vi "Auto_Routine_Deposit.vi"(8 "error in (no error)":errorcluster, 10 "Game Piece":T1, 11 "Position":T2=enum."Middle") -> (0 "error out":errorcluster)   [LabVIEW 2020]
uses:
  Arm/ArmPositionPreset.ctl
  Arm/ArmGamePiecePreset.ctl
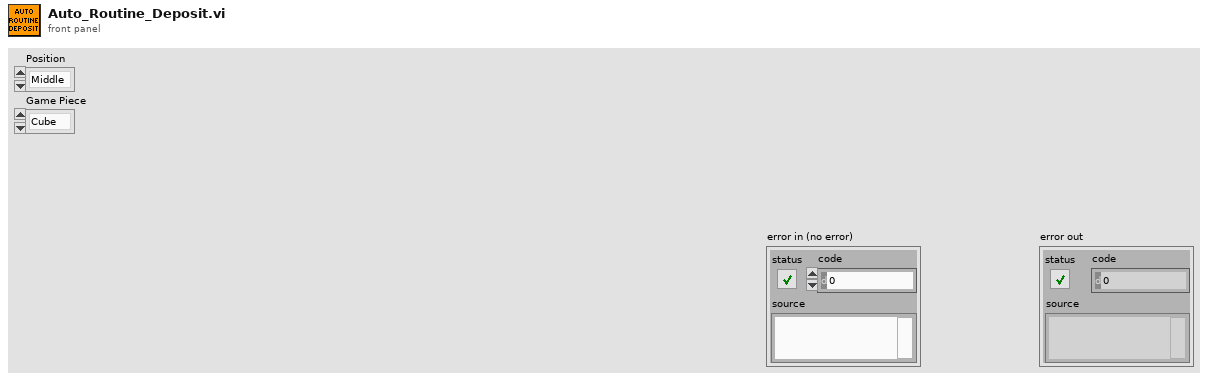
[diagram p1: front panel]
types:
  T1 = typedef "ArmGamePiecePreset.ctl" = enum16{"Cube", "Cone"}
  T2 = typedef "ArmPositionPreset.ctl" = enum16{"Upper", "Lower", "Middle", "Home", "Shelf", "Floor", "HalfFloor", "HalfHome"}
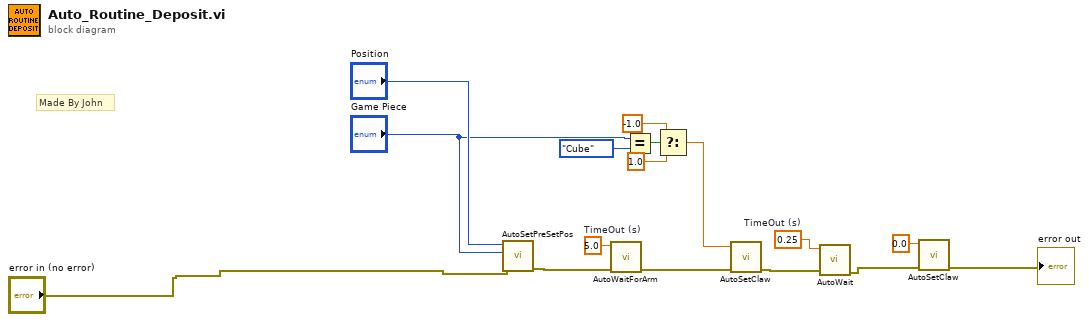
[diagram p0: block diagram]
diagram:
  w16 = 0.25  # TimeOut (s)
  w15 = 5.0  # TimeOut (s)
  # "Made By John"
  n1 = call "AutoSetPreSetPos.vi"("error in (no error)"="error in (no error)", "Game Piece"="Game Piece", "Position"="Position") -> ("error out"=w13:errorcluster)  [unwired: 8 in]
  n2 = call "AutoWaitForArm.vi"("error in (no error)"=w13, "TimeOut (s)"=w15) -> ("error out"=w12:errorcluster)  [unwired: 9 in]
  n3 = Equal?(x="Game Piece", y=ArmGamePiecePreset."Cube") -> (x = y?=w5:bool)
  n4 = Select(t=-1.0, s=w5, f=1.0) -> (s? t:f=w4:dbl)
  n5 = call "AutoSetClaw.vi"("error in (no error)"=w12, "ClawDemand"=w4) -> ("error out"=w11:errorcluster)  [unwired: 9 in]
  n6 = call "AutoWait.vi"("error in (no error)"=w11, "TimeOut (s)"=w16) -> ("error out"=w9:errorcluster)  [unwired: 9 in]
  n7 = call "AutoSetClaw.vi"("error in (no error)"=w9, "ClawDemand"=0.0) -> ("error out"=→"error out":errorcluster)  [unwired: 9 in]
